vi "Sparse To Dense Problem.vi"(8 "error in (no error)":errorcluster, 11 "Sparse Problem":T2) -> (0 "error out":errorcluster, 3 "Dense Problem":T1)   [LabVIEW 2015]
uses:
  LibSVM Sparse/Wrapper API/Controls/svm_problem.ctl
  LibSVM Sparse/Wrapper API/Controls/svm_node.ctl
  LibSVM Dense/Wrapper API/Controls/svmdense_problem.ctl
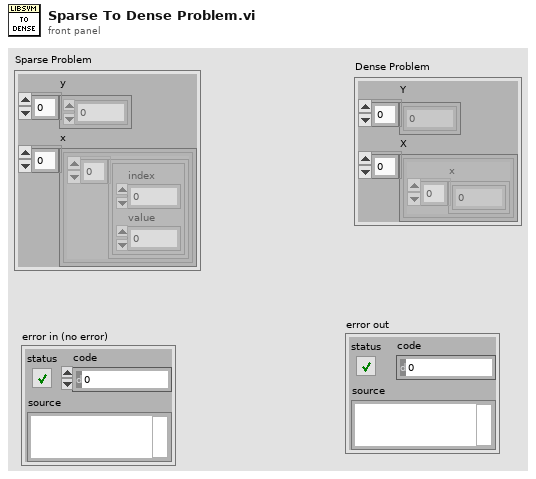
[diagram p1: front panel]
types:
  T1 = typedef "svmdense_problem.ctl" = cluster{"Y":dbl[], "X":cluster{"x":dbl[]}[]}
  T2 = typedef "svm_problem.ctl" = cluster{"y":dbl[], "x":cluster{T3[]}[]}
  T3 = typedef "svm_node.ctl" = cluster{"index":i32, "value":dbl}
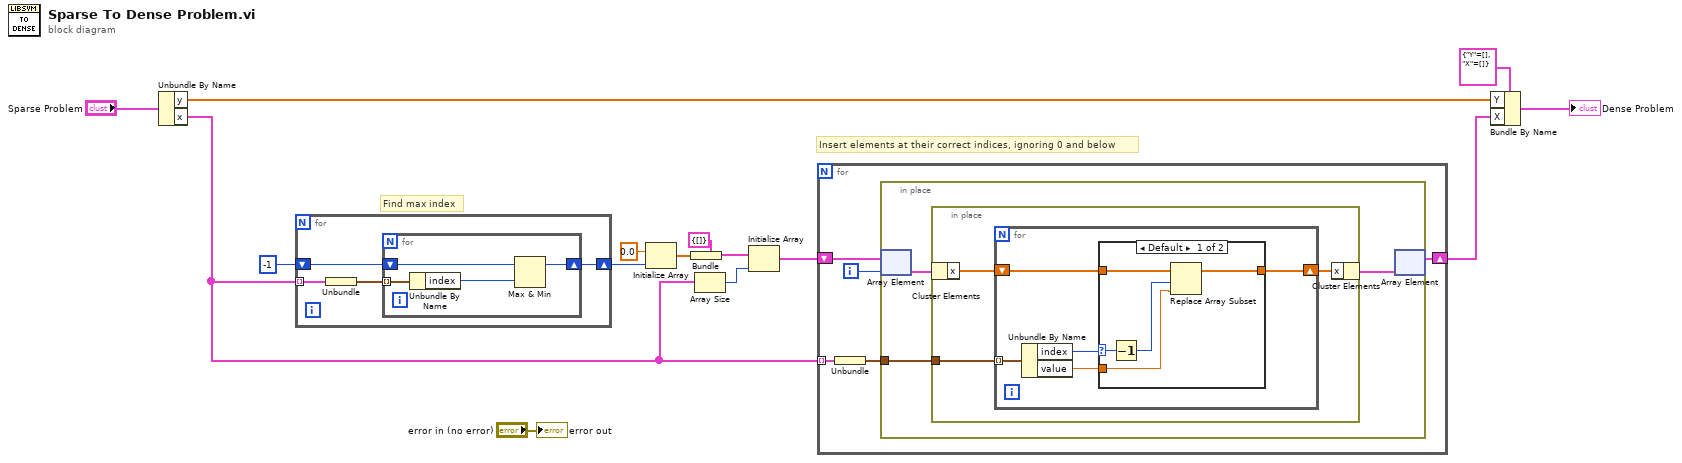
[diagram p0: block diagram]
diagram:
  # "Insert elements at their correct indices, ignoring 0 and below"
  # "Find max index"
  n1 = Unbundle By Name("Sparse Problem") -> ("y"=w13:dbl[], "x"=w6:cluster{T3[]}[])
  n2 = for {
    tunnel: w6 -> [w19] mode=indexing
    shift-right: [w17] -> w10
    shift-left: -1 ("index") -> [w16]
    n3 = Unbundle(w19) -> (w18:T3[])
    n4 = for {
      tunnel: w18 -> [w21] mode=indexing
      shift-right: [w22] -> w17
      shift-left: w16 -> [w23]
      n5 = Unbundle By Name(w21) -> ("index"=w20:i32)
      n6 = Max & Min(x=w23, y=w20) -> (max(x,y)=w22:i32)  [unwired: 1 out]
    }
  }
  n7 = Initialize Array(0.0 ("Numeric"), w10) -> (w9:dbl[])
  n8 = Bundle(cluster=cluster{"x":dbl[]} {"x"=[]}, "x"=w9) -> (w8:cluster{"x":dbl[]})
  n9 = Array Size(array=w6) -> (size(s)=w7:i32)
  n10 = Initialize Array(w8, w7) -> (w5:cluster{"x":dbl[]}[])
  n11 = for {
    tunnel: w6 -> [w28] mode=indexing
    shift-right: [w24] -> w3
    shift-left: w5 -> [w26]
    i -> [w25]
    n12 = Unbundle(w28) -> (w27:T3[])
    n13 = in-place {
      in-place-border: w27 -> [w31]
      n14 = in-place-array #1(w26, w25) -> (w30:cluster{"x":dbl[]})
      n15 = in-place {
        in-place-border: w31 -> [w34]
        n16 = in-place-cluster #2(w30) -> ("x"=w33:dbl[])
        n17 = for {
          shift-right: [w35] -> w32
          shift-left: w33 -> [w37]
          tunnel: w34 -> [w39] mode=indexing
          n18 = Unbundle By Name(w39) -> ("index"=w38:i32, "value"=w36:dbl)
          n19 = case shown="Default" w38 {
            selector: w38 -> [w43 _]
            tunnel: w37 -> [w44 w45]
            tunnel: [w40 w45] -> w35
            tunnel: w36 -> [w41 _]
            frame Default {
              n20 = Decrement(x=w43) -> (x-1=w42:i32)
              n21 = Replace Array Subset(array=w44, new element=w41, index=w42) -> (w40:dbl[])
            }
            frame ..0 {
            }
          }
        }
        n22 = in-place-cluster #2("x"=w32) -> (w29:cluster{"x":dbl[]})
      }
      n23 = in-place-array #1(w29) -> (w24:cluster{"x":dbl[]}[])  [unwired: 1 out]
    }
  }
  n24 = Bundle By Name(cluster=T1 {"Y"=[], "X"=[]} ("Dense Problem"), "Y"=w13, "X"=w3) -> (→"Dense Problem":T1)
  "error out" <- "error in (no error)"
